vi "Wait for spectrometer.vi"(8 "error in (no error)":errorcluster, 10 "milliseconds to wait":u32, 11 "VISA Refnum in":refnum<visa-resource-name>) -> (0 "error out":errorcluster, 2 "SRQ 1 Control Value":u16, 3 "VISA Refnum out":refnum<visa-resource-name>)   [LabVIEW 2021]
uses:
  3fece9f4-d1c8-4801-b2bd-7f9af7cafd55.vi
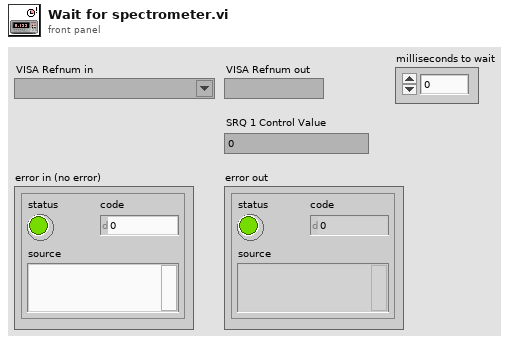
[diagram p1: front panel]
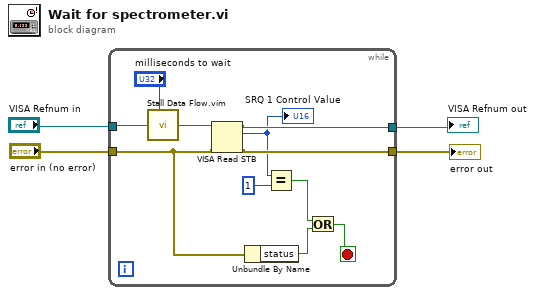
[diagram p0: block diagram]
diagram:
  n1 = while {
    tunnel: "VISA Refnum in" -> [w11]
    tunnel: "error in (no error)" -> [w8]
    tunnel: [w14] -> w2
    tunnel: [w13] -> w3
    stop <- w5 stop-if-true
    n2 = call "Stall Data Flow.vim"("value in"=w11, "milliseconds to wait"="milliseconds to wait") -> ("value out"=w10:refnum<visa-resource-name>)  [unwired: 1 out]
    n3 = VISA Read STB(8:w8, 11:w10) -> (0:w13:errorcluster, 2:w12:u16, 3:w14:refnum<visa-resource-name>)
    "SRQ 1 Control Value" <- w12
    n4 = Unbundle By Name(w8) -> ("status"=w6:bool)
    n5 = Equal?(x=w12, y=u16 1) -> (x = y?=w7:bool)
    n6 = Or(x=w7, y=w6) -> (x .or. y?=w5:bool)
  }
  "error out" <- w3
  "VISA Refnum out" <- w2
